vi "spring - move item.vi"(7 "tree ref":refnum<vi>, 8 "error in (no error)":errorcluster, 9 "position (0=just below parent etc.)":i32, 10 "parent tag":string, 11 "tag":string) -> (0 "error out":errorcluster)   [LabVIEW 2014]
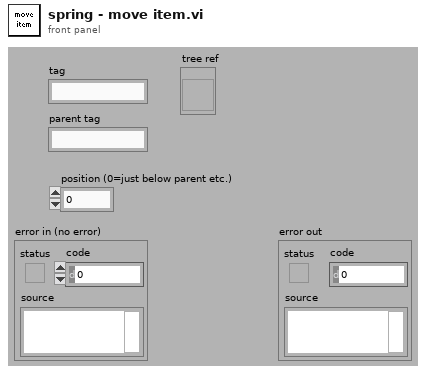
[diagram p1: front panel]
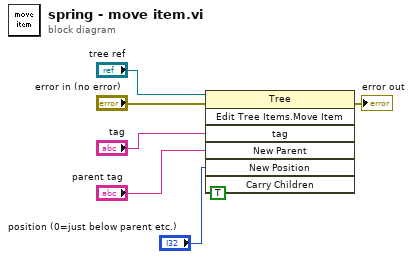
[diagram p0: block diagram]
diagram:
  n1 = invoke class="Tree" method="Edit Tree Items.Move Item"(reference="tree ref", error in="error in (no error)", "tag"="tag", "New Parent"="parent tag", "New Position"="position (0=just below parent etc.)", "Carry Children"=TRUE) -> (error out=→"error out":errorcluster)  [unwired: 1 in, 6 out]
